vi "SRV_Get Data Subset for Sensors Config Display.vi"(0 "All Sensors Config":T1[](array[typedef]) {"Register" format="%.0x"; "I2C Address" format="%.0x"; "Sample Period (ms)" min=10 max=60000 step=1; "Digital Mask" format="%.0x"; "Channel" format="%.0x"}, 11 "error in (no error)":errorcluster, 12 "Row Start Index":i32, 13 "Number of Rows to Display (3)":i32=3) -> (4 "All Sensors Config dup":T1[](array[typedef]) {"Register" format="%.0x"; "I2C Address" format="%.0x"; "Sample Period (ms)" min=10 max=60000 step=1; "Digital Mask" format="%.0x"; "Channel" format="%.0x"}, 6 "Sensors Config GUI":T9={"Sensor Index 0"={"Name"="Button xx", "A/D"=enum."Analog", "I2C Address"=0, "Register"=0, "Channel"=0, "Digital Mask"=0, "Units"="", "Sampling Mode"=enum."Polled", "Sample Period (ms)"=1000, "Formula"="", "Sensor View Config"={"Sensor Name"=enum."Gauge 01", "Minimum"=0.0, "Maximum"=10.0}, "Active"=FALSE, "PicoC Shared Var Type"=enum."Integer", "Index"=0, "Stream Multiple?"=FALSE, "Index End"=255, "Bytes"=enum."1 Byte", "Source Sensor Name"="", "Repeat Start"=FALSE, "Integer Word Type"=enum."Unsigned", "Byte Swap"=FALSE}, "Sensor Index 1"={"Name"="Button xx", "A/D"=enum."Analog", "I2C Address"=0, "Register"=0, "Channel"=0, "Digital Mask"=0, "Units"="", "Sampling Mode"=enum."Polled", "Sample Period (ms)"=1000, "Formula"="", "Sensor View Config"={"Sensor Name"=enum."Gauge 01", "Minimum"=0.0, "Maximum"=10.0}, "Active"=FALSE, "PicoC Shared Var Type"=enum."Integer", "Index"=0, "Stream Multiple?"=FALSE, "Index End"=255, "Bytes"=enum."1 Byte", "Source Sensor Name"="", "Repeat Start"=FALSE, "Integer Word Type"=enum."Unsigned", "Byte Swap"=FALSE}, "Sensor Index 2"={"Name"="Button xx", "A/D"=enum."Analog", "I2C Address"=0, "Register"=0, "Channel"=0, "Digital Mask"=0, "Units"="", "Sampling Mode"=enum."Polled", "Sample Period (ms)"=1000, "Formula"="", "Sensor View Config"={"Sensor Name"=enum."Gauge 01", "Minimum"=0.0, "Maximum"=10.0}, "Active"=FALSE, "PicoC Shared Var Type"=enum."Integer", "Index"=0, "Stream Multiple?"=FALSE, "Index End"=255, "Bytes"=enum."1 Byte", "Source Sensor Name"="", "Repeat Start"=FALSE, "Integer Word Type"=enum."Unsigned", "Byte Swap"=FALSE}} {"Sensor Index 2"."Register" format="%.0x"; "Sensor Index 2"."I2C Address" format="%.0x"; "Sensor Index 2"."Sample Period (ms)" min=10 max=60000 step=1; "Sensor Index 2"."Digital Mask" format="%.0x"; "Sensor Index 2"."Channel" format="%.0x"; "Sensor Index 1"."Register" format="%.0x"; "Sensor Index 1"."I2C Address" format="%.0x"; "Sensor Index 1"."Sample Period (ms)" min=10 max=60000 step=1; "Sensor Index 1"."Digital Mask" format="%.0x"; "Sensor Index 1"."Channel" format="%.0x"; "Sensor Index 0"."Register" format="%.0x"; "Sensor Index 0"."I2C Address" format="%.0x"; "Sensor Index 0"."Sample Period (ms)" min=10 max=60000 step=1; "Sensor Index 0"."Digital Mask" format="%.0x"; "Sensor Index 0"."Channel" format="%.0x"}, 15 "error out":errorcluster)   [LabVIEW 2014]
doc: "Author: Mike Schultz (LogicPD, Inc)"
uses:
  SRV_Sensor Config Cluster.ctl
  SRV_Sensor Analog-Digital.ctl
  SRV_Sensor Sampling Mode.ctl
  SRV_Sensor View Config Cluster.ctl
  SRV_Sensors Names.ctl
  SRV_Sensor PicoC Shared Var Type.ctl
  SRV_Sensor Number of Bytes.ctl
  SRV_Sensor Integer Word Type.ctl
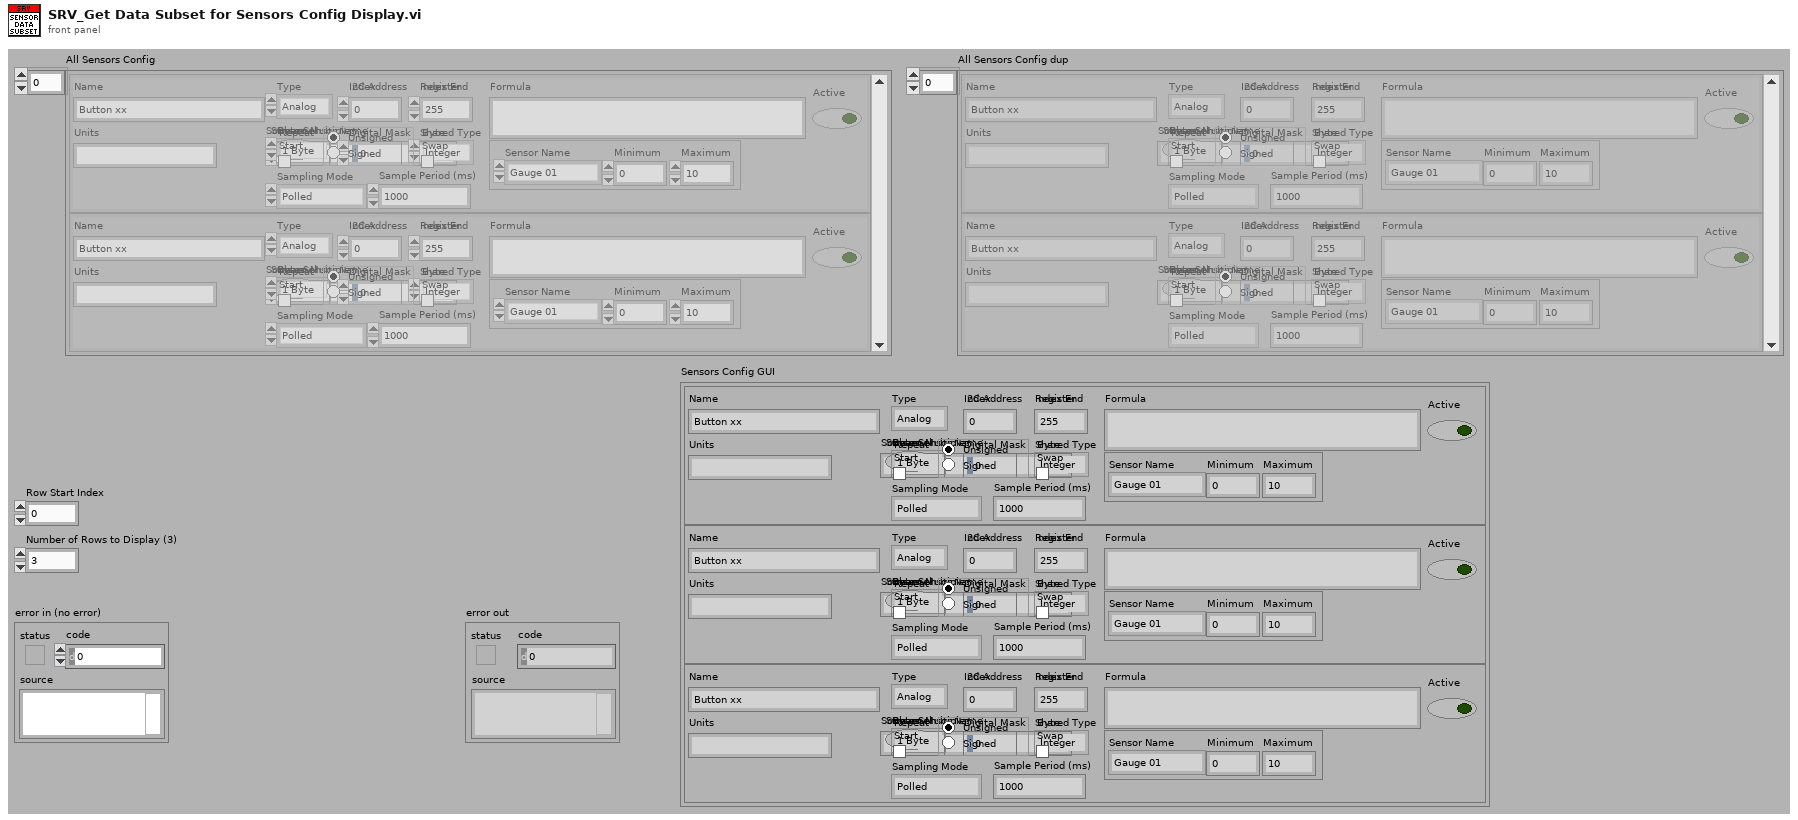
[diagram p1: front panel]
types:
  T1 = typedef "SRV_Sensor Config Cluster.ctl" = cluster{"Name":string, "A/D":T2, "I2C Address":u8, "Register":u8, "Channel":u8, "Digital Mask":u16, "Units":string, "Sampling Mode":T3, "Sample Period (ms)":u32, "Formula":string, "Sensor View Config":T4, "Active":bool, "PicoC Shared Var Type":T6, "Index":u8, "Stream Multiple?":bool, "Index End":u8, "Bytes":T7, "Source Sensor Name":string, "Repeat Start":bool, "Integer Word Type":T8, "Byte Swap":bool}
  T2 = typedef "SRV_Sensor Analog-Digital.ctl" = enum16{"Digital", "Analog", "PicoC Shared", "Calculated"}
  T3 = typedef "SRV_Sensor Sampling Mode.ctl" = enum16{"Polled", "Streaming"}
  T4 = typedef "SRV_Sensor View Config Cluster.ctl" = cluster{"Sensor Name":T5, "Minimum":dbl, "Maximum":dbl}
  T5 = typedef "SRV_Sensors Names.ctl" = enum16{"Gauge 01", "Gauge 02", "Gauge 03", "Gauge 04", "Meter 01", "Meter 02", "Meter 03", "Meter 04", "Numeric 01", "Numeric 02", "Numeric 03", "Numeric 04", "Numeric 05", "Numeric 06", "Numeric 07", "Numeric 08", "Boolean 01", "Boolean 02", "Boolean 03", "Boolean 04", "Boolean 05", "Boolean 06", "Boolean 07", "Boolean 08", "Boolean 09", "Boolean 10", "Boolean 11", "Boolean 12", "Boolean 13", "Boolean 14", "Boolean 15", "Boolean 16", "Boolean 17", "Boolean 18", "Boolean 19", "Boolean 20", "Boolean 21", "Boolean 22", "Boolean 23", "Boolean 24", "Boolean 25", "Boolean 26", "Boolean 27", "Boolean 28", "Boolean 29", "Boolean 30", "Boolean 31", "Boolean 32"}
  T6 = typedef "SRV_Sensor PicoC Shared Var Type.ctl" = enum16{"String", "Integer", "Float"}
  T7 = typedef "SRV_Sensor Number of Bytes.ctl" = enum16{"1 Byte", "2 Bytes"}
  T8 = typedef "SRV_Sensor Integer Word Type.ctl" = enum32{"Unsigned", "Signed"}
  T9 = cluster{"Sensor Index 0":T1, "Sensor Index 1":T1, "Sensor Index 2":T1}
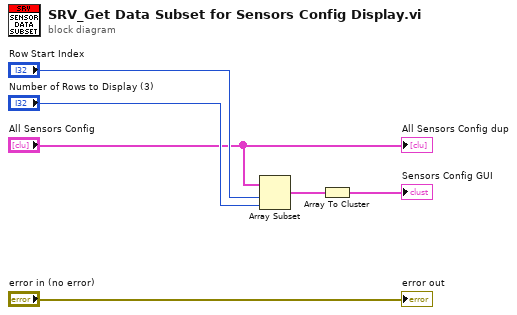
[diagram p0: block diagram]
diagram:
  n1 = Array Subset(array="All Sensors Config", index="Row Start Index", length="Number of Rows to Display (3)") -> (w2:T1[])
  n2 = Array To Cluster(array=w2) -> (cluster=→"Sensors Config GUI":cluster{"[0]":T1, "[1]":T1, "[2]":T1})
  "All Sensors Config dup" <- "All Sensors Config"
  "error out" <- "error in (no error)"
